vi "Debuger.vi"(11 "DevControl输入":refnum<class "DevControl.lvclass">=refnum) -> ()   [LabVIEW 2012]
uses:
  Fun/Dev/DevControl.lvclass
  Libs/Serial/Serial.lvclass
  Fun/Dev/SupportVi/DevState.ctl
panel:
  in  "确定按钮":bool
  in  "ßxÖÐ":bool
  in  "Send":bool
  in  "DevCmd":u8(ring)=34 items=["Red"=66, "Green"=65, "TurnOn"=49, "Shutdown"=48, "GetESD"=34]
  in  "AllDev":cluster{"Addr":u8, "ÑbÖÃ î‘B":T1, "ßxÖÐ":bool}[](array[cluster])
  in  "Scan":bool
  in  "Stop":u8
  in  "Start":u8
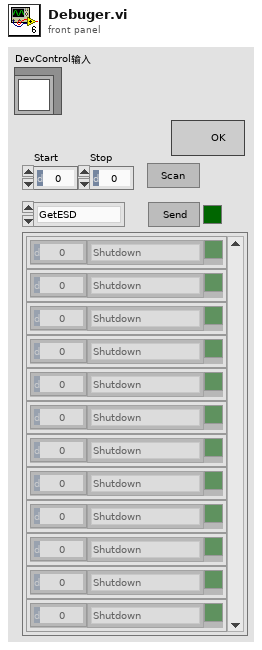
[diagram p1: front panel]
types:
  T1 = typedef "DevControl.lvclass/DevState.ctl" = enum16{"Shutdown", "PASS", "FAIL", "Idle", "Noresponse"}
  T2 = cluster{"Addr":i32, "ÑbÖÃ î‘B":T1, "ßxÖÐ":bool}[]
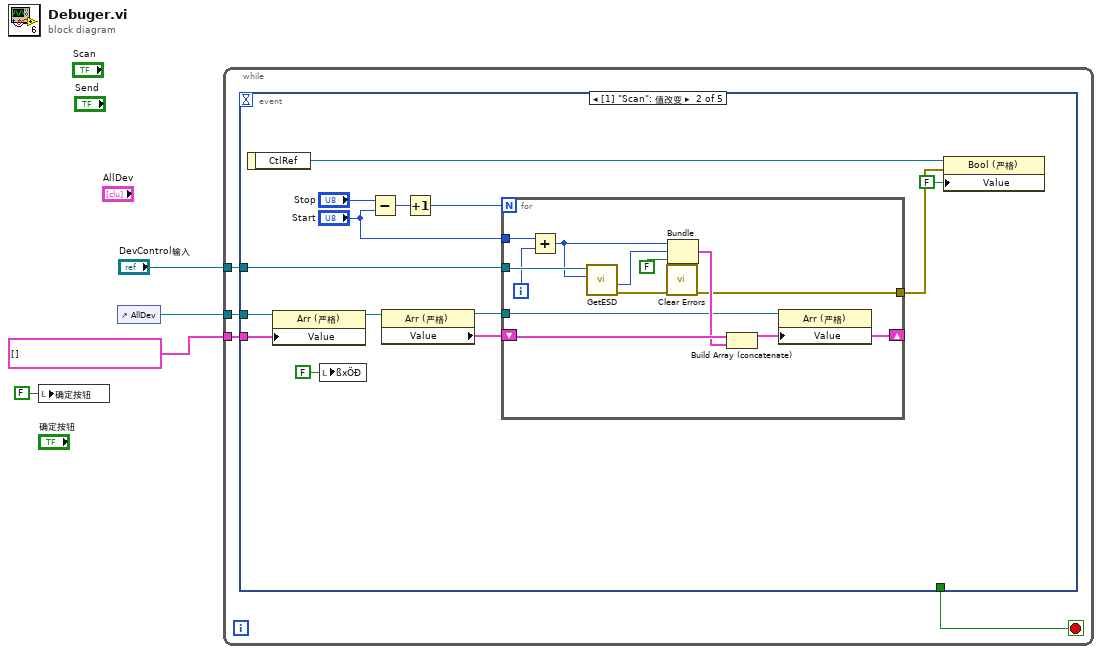
[diagram p0: block diagram]
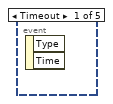
[diagram p2: hidden frame]
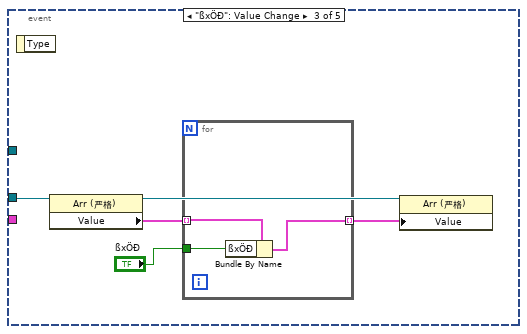
[diagram p3: hidden frame]
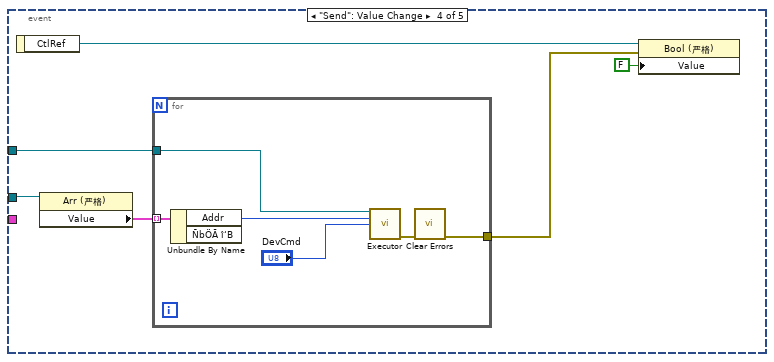
[diagram p4: hidden frame]
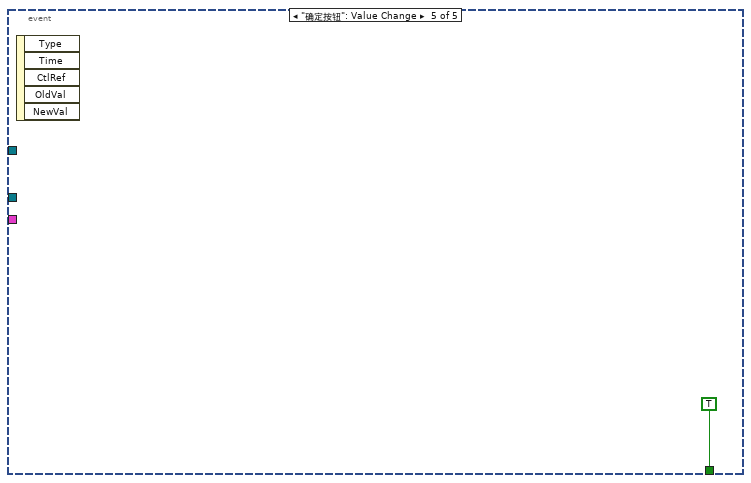
[diagram p5: hidden frame]
diagram:
  n1 = local write "确定按钮"(FALSE ("确定按钮")) -> ()
  n2 = control-ref of="AllDev"() -> (w3:refnum<vi>)
  n3 = while {
    tunnel: "DevControl输入" -> [w8]
    tunnel: w3 -> [w7]
    tunnel: cluster{"Addr":u8, "ÑbÖÃ î‘B":T1, "ßxÖÐ":bool}[] [] ("AllDev") -> [w6]
    stop <- w5 stop-if-true
    n4 = event shown="[1] \"Scan\": 值改变" {
      selector: _ -> [_ _ _ _ _]
      dyn-events: _ -> [_ _ _ _ _]
      timeout: _ -> [_ _ _ _ _]
      tunnel: w8 -> [_ w19 _ w46 _]
      tunnel: w7 -> [_ w17 w39 w48 _]
      tunnel: w6 -> [_ w16 _ _ _]
      tunnel: [_ _ _ _ TRUE] -> w5
      event Timeout {
        n5 = event-data() -> ()  [unwired: 1 in, 2 out]
      }
      event "Scan": Value Change {
        n6 = event-data() -> ("CtlRef"=w12:refnum<vi>)  [unwired: 1 in]
        n7 = property class="Arr (严格)"(reference=w17, "Value"=w16) -> (reference out=w15:refnum<vi>)  [unwired: 1 in, 1 out]
        n8 = local write "ßxÖÐ"(FALSE ("ßxÖÐ")) -> ()
        n9 = Subtract(x="Stop", y="Start") -> (x-y=w20:u8)
        n10 = property class="Arr (严格)"(reference=w15) -> (reference out=w13:refnum<vi>, "Value"=w14:cluster{"Addr":u8, "ÑbÖÃ î‘B":T1, "ßxÖÐ":bool}[])  [unwired: 1 in, 1 out]
        n11 = Increment(x=w20) -> (x+1=w21:u8)
        n12 = for {
          N: w21 -> [_]
          tunnel: w19 -> [w34]
          tunnel: "Start" -> [w33]
          tunnel: w13 -> [w25]
          shift-right: [w24] -> _
          shift-left: w14 -> [w27]
          tunnel: [w23] -> w11
          i -> [w32]
          n13 = Add(x=w33, y=w32) -> (x+y=w31:i32)
          n14 = call-dynamic "GetESD.vi"("Addr"=w31, "DevControl 输入"=w34) -> ("error out"=w29:errorcluster, "ÑbÖÃ î‘B"=w30:T1)  [unwired: 7 in, 1 out]
          n15 = call <vilib>:"Clear Errors.vi"("error in (no error)"=w29) -> ("error out"=w23:errorcluster)  [unwired: 6 in]
          n16 = Bundle(w31, "ÑbÖÃ î‘B"=w30, FALSE) -> (w26:cluster{i32, "ÑbÖÃ î‘B":T1, bool})  [unwired: 1 in]
          n17 = Build Array (concatenate)(w27, w26) -> (w24:T2)
          n18 = property class="Arr (严格)"(reference=w25, "Value"=w24) -> ()  [unwired: 1 in, 2 out]
        }
        n19 = property class="Bool (严格)"(reference=w12, error in=w11, "Value"=FALSE ("值")) -> ()  [unwired: 2 out]
      }
      event "ßxÖÐ": Value Change {
        n20 = event-data() -> ()  [unwired: 1 in, 1 out]
        n21 = property class="Arr (严格)"(reference=w39) -> (reference out=w37:refnum<vi>, "Value"=w38:cluster{"Addr":u8, "ÑbÖÃ î‘B":T1, "ßxÖÐ":bool}[])  [unwired: 1 in, 1 out]
        n22 = for {
          tunnel: w38 -> [w42] mode=indexing
          tunnel: [w41] -> w36 mode=indexing
          tunnel: "ßxÖÐ" -> [w40]
          n23 = Bundle By Name(cluster=w42, "ßxÖÐ"=w40) -> (w41:cluster{"Addr":u8, "ÑbÖÃ î‘B":T1, "ßxÖÐ":bool})
        }
        n24 = property class="Arr (严格)"(reference=w37, "Value"=w36) -> ()  [unwired: 1 in, 2 out]
      }
      event "Send": Value Change {
        n25 = event-data() -> ("CtlRef"=w45:refnum<vi>)  [unwired: 1 in]
        n26 = property class="Arr (严格)"(reference=w48) -> ("Value"=w47:cluster{"Addr":u8, "ÑbÖÃ î‘B":T1, "ßxÖÐ":bool}[])  [unwired: 1 in, 2 out]
        n27 = for {
          tunnel: w47 -> [w54] mode=indexing
          tunnel: w46 -> [w52]
          tunnel: [w49] -> w44
          n28 = Unbundle By Name(w54) -> ("Addr"=w53:u8)  [unwired: 1 out]
          n29 = call-dynamic "Executor.vi"("DevControl 输入"=w52, "Addr"=w53, "DevCmd"="DevCmd") -> ("error out"=w50:errorcluster)  [unwired: 10 in, 2 out]
          n30 = call <vilib>:"Clear Errors.vi"("error in (no error)"=w50) -> ("error out"=w49:errorcluster)  [unwired: 6 in]
        }
        n31 = property class="Bool (严格)"(reference=w45, error in=w44, "Value"=FALSE ("值")) -> ()  [unwired: 2 out]
      }
      event "确定按钮": Value Change {
        n32 = event-data() -> ()  [unwired: 1 in, 5 out]
      }
    }
  }
